vi "Demo Control.vi"() -> ()   [LabVIEW 2020]
panel:
  in  "System Config Status":T1
  in  "Sequencing":T2={"Sequences"=[], "Unload All"=FALSE, "Abort All"=FALSE, "Loaded, Good CRC"=13816530, "Sequence Error"=16744319, "Loaded, CRC Mismatch"=16777142, "Running, Good CRC"=11730866, "Unloaded"=7171459, "Running, CRC Mismatch"=10530559}
  in  "Logging Control":T3
  # "Config Status"
  # "Ver"
  # "Hash"
  # "Sequence"
  # "State"
  # "State Time"
  # "Seq Time"
  # "Started"
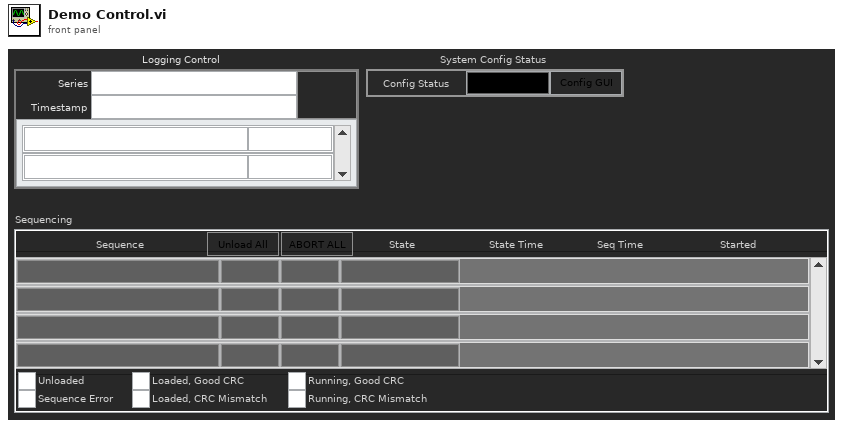
[diagram p1: front panel]
types:
  T1 = cluster{"Status Color":u32, "Status String":string, "Config GUI":bool, "Status":cluster{"Node Name":string, "Node Color":u32, "Version Color":u32, "Hash Color":u32}[]}
  T2 = cluster{"Sequences":cluster{"Name Color":u32, "Name":string, "Btn 1 Color":u32, "Btn 1 Text":string, "Btn 2 Color":u32, "Btn 2 Text":string, "Status Color":u32, "Status":string, "State Time":string, "Started":string, "Seq Time":string, "Btn 1":bool, "Btn 2":bool, "Btn Name":bool}[], "Unload All":bool, "Abort All":bool, "Loaded, Good CRC":u32, "Sequence Error":u32, "Loaded, CRC Mismatch":u32, "Running, Good CRC":u32, "Unloaded":u32, "Running, CRC Mismatch":u32}
  T3 = cluster{"Series":string, "Timestamp":string, "Log Button":bool, "Status":cluster{"Node":string, "Node Color":u32, "State":string}[]}
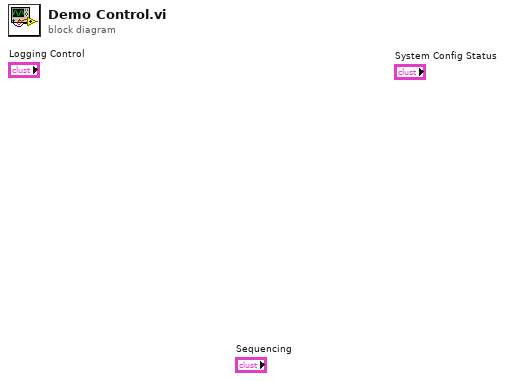
[diagram p0: block diagram]
diagram:
